vi "Data checking for mode (SILAR_Data checking).vi"(0 "Режим погружения подложки":u16(ring)=1 items=["Частичное", "Полное"], 1 "Кол-во используемых растворов":i32(ring)=2 items=["Один"=1, "Два"=2, "Три"=3, "Четыре"=4], 5 "Кол-во жидкости в каждом стакане (мм)":dbl[](array[numeric])=[55.0, 55.0, 55.0, 55.0], 7 "Высота подложки":dbl, 9 "Глубина погружения в раствор":dbl[](array[numeric])=[55.0, 55.0, 55.0, 55.0], 11 "Высота стакана":dbl) -> (3 "1":i16, 4 "2":i16, 6 "3":i16, 8 "4":i16, 10 "5":i16, 14 "7":i16, 15 "6":i16)   [LabVIEW 2016]
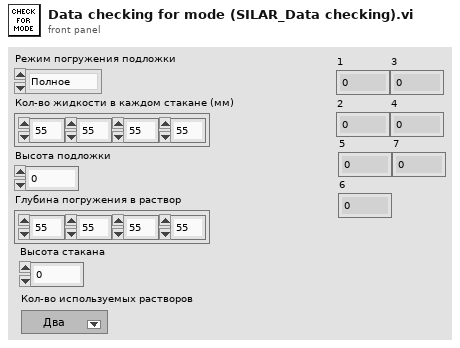
[diagram p1: front panel]
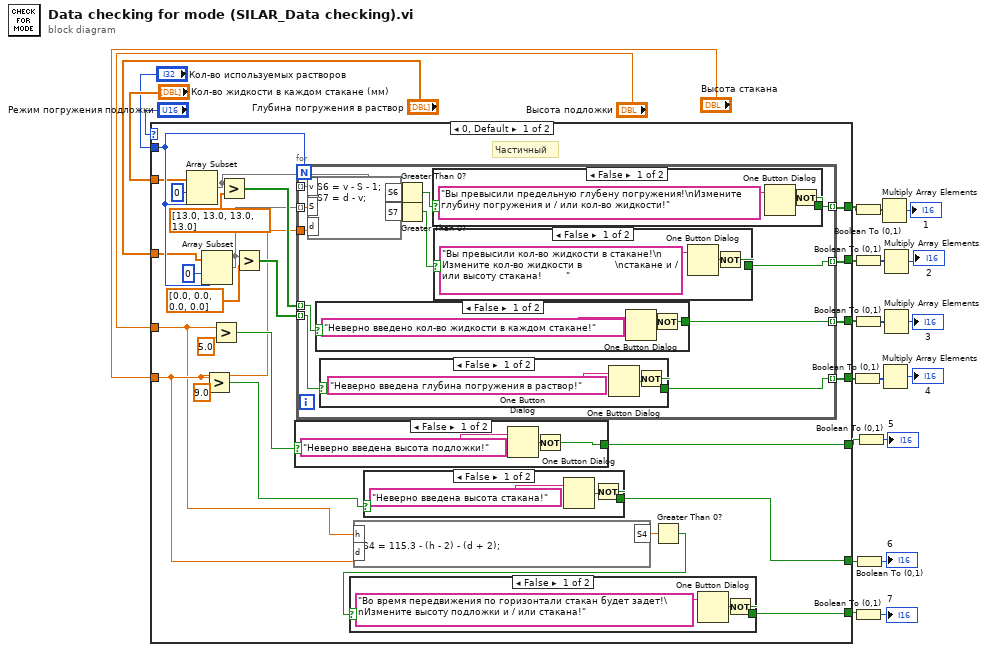
[diagram p0: block diagram]
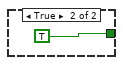
[diagram p2: hidden frame]
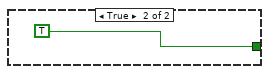
[diagram p3: hidden frame]
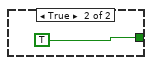
[diagram p4: hidden frame]
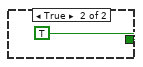
[diagram p5: hidden frame]
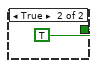
[diagram p6: hidden frame]
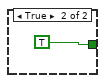
[diagram p7: hidden frame]
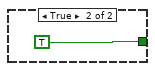
[diagram p8: hidden frame]
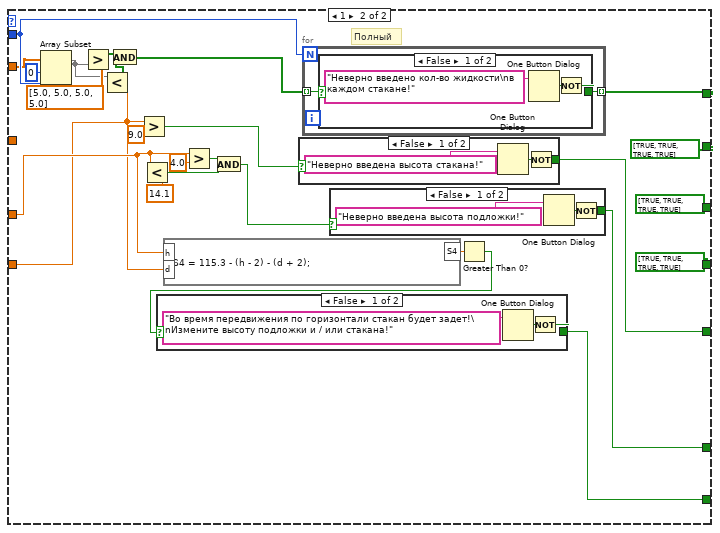
[diagram p9: hidden frame]
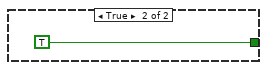
[diagram p10: hidden frame]
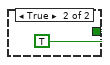
[diagram p11: hidden frame]
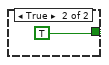
[diagram p12: hidden frame]
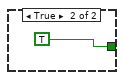
[diagram p13: hidden frame]
diagram:
  n1 = case shown="0, Default" "Режим погружения подложки" {
    tunnel: "Кол-во используемых растворов" -> [w47 w113]
    tunnel: [w49 w114] -> w18
    tunnel: [w42 w115] -> w14
    tunnel: [w43 w116] -> w15
    tunnel: [w36 bool[] [TRUE, TRUE, TRUE, TRUE]] -> w19
    tunnel: [w35 bool[] [TRUE, TRUE, TRUE, TRUE]] -> w16
    tunnel: [w34 bool[] [TRUE, TRUE, TRUE, TRUE]] -> w17
    tunnel: [w33 w99] -> w24
    tunnel: "Кол-во жидкости в каждом стакане (мм)" -> [w28 w94]
    tunnel: "Глубина погружения в раствор" -> [w27 _]
    tunnel: "Высота подложки" -> [w25 w93]
    tunnel: "Высота стакана" -> [w26 w92]
    frame 0, Default {
      # "Частичный"
      n2 = Array Subset(array=w28, index=0, length=w47) -> (w30:dbl[])
      n3 = Array Subset(array=w27, index=0, length=w47) -> (w31:dbl[])
      n4 = Greater?(x=w26, y=9.0) -> (0:w37:bool)
      n5 = Greater?(x=w25, y=5.0) -> (0:w44:bool)
      n6 = Greater?(x=w30, y=dbl[] [13.0, 13.0, 13.0, 13.0]) -> (0:w39:bool[])
      n7 = Greater?(x=w31, y=dbl[] [0.0, 0.0, 0.0, 0.0]) -> (0:w38:bool[])
      n8 = case shown="False" w44 {
        tunnel: [w51 TRUE] -> w43
        frame False {
          n9 = One Button Dialog(message="Неверно введена высота подложки!") -> (true=w52:bool)  [unwired: 1 in]
          n10 = Not(x=w52) -> (.not. x?=w51:bool)
        }
        frame True {
        }
      }
      n11 = for {
        N: w47 -> [_]
        tunnel: [w66] -> w49 mode=indexing
        tunnel: w30 -> [w75] mode=indexing
        tunnel: w31 -> [w74] mode=indexing
        tunnel: w26 -> [w72]
        tunnel: w39 -> [w67] mode=indexing
        tunnel: w38 -> [w68] mode=indexing
        tunnel: [w65] -> w36 mode=indexing
        tunnel: [w63] -> w35 mode=indexing
        tunnel: [w64] -> w34 mode=indexing
        n12 = formula code="S6 = v - S - 1;\nS7 = d - v;"("v"=w75, "S"=w74, "d"=w72) -> ("S6"=w73:dbl, "S7"=w71:dbl)
        n13 = case shown="False" w67 {
          tunnel: [w80 TRUE] -> w64
          frame False {
            n14 = One Button Dialog(message="Неверно введено кол-во жидкости в каждом стакане!") -> (true=w81:bool)  [unwired: 1 in]
            n15 = Not(x=w81) -> (.not. x?=w80:bool)
          }
          frame True {
          }
        }
        n16 = case shown="False" w68 {
          tunnel: [w76 TRUE] -> w63
          frame False {
            n17 = One Button Dialog(message="Неверно введена глубина погружения в раствор!") -> (true=w77:bool)  [unwired: 1 in]
            n18 = Not(x=w77) -> (.not. x?=w76:bool)
          }
          frame True {
          }
        }
        n19 = Greater Than 0?(x=w73) -> (x > 0?=w69:bool)
        n20 = Greater Than 0?(x=w71) -> (x > 0?=w70:bool)
        n21 = case shown="False" w69 {
          tunnel: [w88 TRUE] -> w66
          frame False {
            n22 = One Button Dialog(message="Вы превысили предельную глубену погружения!\nИзмените глубину погружения и / или кол-во жидкости!") -> (true=w89:bool)  [unwired: 1 in]
            n23 = Not(x=w89) -> (.not. x?=w88:bool)
          }
          frame True {
          }
        }
        n24 = case shown="False" w70 {
          tunnel: [w84 TRUE] -> w65
          frame False {
            n25 = One Button Dialog(message="Вы превысили кол-во жидкости в стакане!\n  Измените кол-во жидкости в           \nстакане и / или высоту стакана!        ") -> (true=w85:bool)  [unwired: 1 in]
            n26 = Not(x=w85) -> (.not. x?=w84:bool)
          }
          frame True {
          }
        }
      }
      n27 = formula code="S4 = 115.3 - (h - 2) - (d + 2);"("h"=w25, "d"=w26) -> ("S4"=w46:dbl)
      n28 = case shown="False" w37 {
        tunnel: [w59 TRUE] -> w42
        frame False {
          n29 = One Button Dialog(message="Неверно введена высота стакана!") -> (true=w60:bool)  [unwired: 1 in]
          n30 = Not(x=w60) -> (.not. x?=w59:bool)
        }
        frame True {
        }
      }
      n31 = Greater Than 0?(x=w46) -> (x > 0?=w29:bool)
      n32 = case shown="False" w29 {
        tunnel: [w55 TRUE] -> w33
        frame False {
          n33 = One Button Dialog(message="Во время передвижения по горизонтали стакан будет задет!\nИзмените высоту подложки и / или стакана!") -> (true=w56:bool)  [unwired: 1 in]
          n34 = Not(x=w56) -> (.not. x?=w55:bool)
        }
        frame True {
        }
      }
    }
    frame 1 {
      # "Полный"
      n35 = Array Subset(array=w94, index=0, length=w113) -> (w108:dbl[])
      n36 = Greater?(x=w108, y=dbl[] [5.0, 5.0, 5.0, 5.0] ("x")) -> (0:w107:bool[])
      n37 = Less?(x=w108, y=w92) -> (x < y?=w96:bool[])
      n38 = And(x=w107, y=w96) -> (x .and. y?=w97:bool[])
      n39 = Greater?(x=w92, y=9.0) -> (0:w98:bool)
      n40 = Less?(x=w93, y=14.1) -> (x < y?=w102:bool)
      n41 = formula code="S4 = 115.3 - (h - 2) - (d + 2);"("h"=w93, "d"=w92) -> ("S4"=w100:dbl)
      n42 = Greater?(x=w93, y=4.0) -> (0:w103:bool)
      n43 = And(x=w103, y=w102) -> (x .and. y?=w101:bool)
      n44 = case shown="False" w98 {
        tunnel: [w122 TRUE] -> w116
        frame False {
          n45 = One Button Dialog(message="Неверно введена высота стакана!") -> (true=w123:bool)  [unwired: 1 in]
          n46 = Not(x=w123) -> (.not. x?=w122:bool)
        }
        frame True {
        }
      }
      n47 = for {
        N: w113 -> [_]
        tunnel: [w131] -> w114 mode=indexing
        tunnel: w97 -> [w130] mode=indexing
        n48 = case shown="False" w130 {
          tunnel: [w132 TRUE] -> w131
          frame False {
            n49 = One Button Dialog(message="Неверно введено кол-во жидкости\nв каждом стакане!") -> (true=w133:bool)  [unwired: 1 in]
            n50 = Not(x=w133) -> (.not. x?=w132:bool)
          }
          frame True {
          }
        }
      }
      n51 = case shown="False" w101 {
        tunnel: [w126 TRUE] -> w115
        frame False {
          n52 = One Button Dialog(message="Неверно введена высота подложки!") -> (true=w127:bool)  [unwired: 1 in]
          n53 = Not(x=w127) -> (.not. x?=w126:bool)
        }
        frame True {
        }
      }
      n54 = Greater Than 0?(x=w100) -> (x > 0?=w95:bool)
      n55 = case shown="False" w95 {
        tunnel: [w118 TRUE] -> w99
        frame False {
          n56 = One Button Dialog(message="Во время передвижения по горизонтали стакан будет задет!\nИзмените высоту подложки и / или стакана!") -> (true=w119:bool)  [unwired: 1 in]
          n57 = Not(x=w119) -> (.not. x?=w118:bool)
        }
        frame True {
        }
      }
    }
  }
  n58 = Boolean To (0,1)(Boolean=w16) -> (0, 1=w13:i16[])
  n59 = Boolean To (0,1)(Boolean=w18) -> (0, 1=w10:i16[])
  n60 = Boolean To (0,1)(Boolean=w19) -> (0, 1=w11:i16[])
  n61 = Boolean To (0,1)(Boolean=w17) -> (0, 1=w12:i16[])
  n62 = Boolean To (0,1)(Boolean=w24) -> (0, 1=→"7":i16)
  n63 = Boolean To (0,1)(Boolean=w14) -> (0, 1=→"6":i16)
  n64 = Boolean To (0,1)(Boolean=w15) -> (0, 1=→"5":i16)
  n65 = Multiply Array Elements(1:w10) -> (0:→"1":i16)
  n66 = Multiply Array Elements(1:w13) -> (0:→"4":i16)
  n67 = Multiply Array Elements(1:w11) -> (0:→"2":i16)
  n68 = Multiply Array Elements(1:w12) -> (0:→"3":i16)
